vi "Initialise.vi"(8 "error in (no error)":errorcluster, 10 "Message in":refnum<class "InitialiseMessage.lvclass">, 11 "Tomo in":refnum<class "Invivo_Tomo.lvclass">) -> (0 "error out":errorcluster, 3 "Tomo out":refnum<class "Invivo_Tomo.lvclass">)   [LabVIEW 2012, in "Invivo_Tomo.lvclass"]
doc: "This method is called when an initialise message is received. It mainly initialises the RabbitMQ connectivity. \n\nOverride this method when your component needs special initialisation (e.g. of software or hardware resources). In that case, don't forget to call the parent for proper implementation. If your component owns subcomponents, they count as resources, so you have to initialise them by calling their own initialise functions"
uses:
  Invivo_Tomo.lvclass
  <vilib>/Distrio/Murmex/InitialiseMessage/InitialiseMessage.lvclass
  <vilib>/Distrio/Murmex/Murmex/Murmex.lvclass
  Current activity.ctl
panel:
  # "This method is called when the INTIALISE\ntrigger is sent. \n\nOverride this method when your component needs to\nrespond to this trigger. \n\nCall parent for proper implementation"
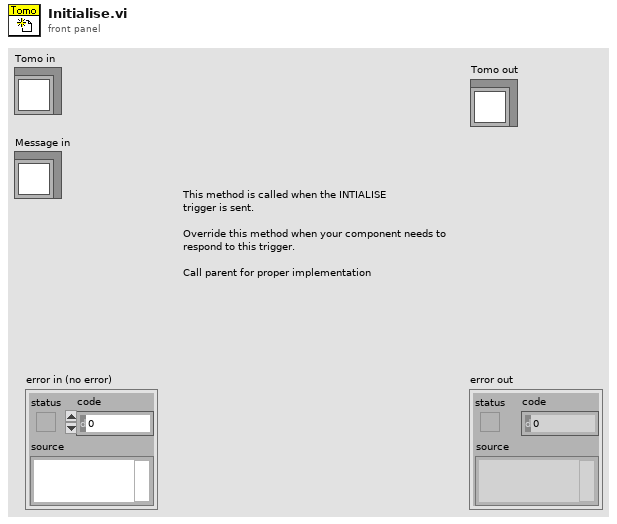
[diagram p1: front panel]
types:
  T1 = typedef "Invivo_Tomo.lvclass/Current activity.ctl" = enum16{"Idle", "Inter-stack motion", "Autofocus", "Stack acquisition"}
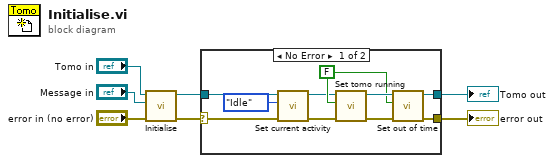
[diagram p0: block diagram]
diagram:
  n1 = call-parent "Initialise.vi"("error in (no error)"="error in (no error)", "Message in"="Message in", "Murmex in"="Tomo in") -> ("error out"=w4:errorcluster, "Murmex out"=w3:refnum<class "Invivo_Tomo.lvclass">)  [unwired: 7 in]
  n2 = case shown="No Error" w4 {
    selector: w4 -> [w10 w18]
    tunnel: w3 -> [w9 w19]
    tunnel: [w16 w18] -> w2
    tunnel: [w14 w19] -> w1
    frame No Error {
      w13 = FALSE ("is acquiring?")
      n3 = call-dynamic "Set current activity.vi"("error in (no error)"=w10, "Current activity"=Current_activity."Idle", "Tomo in"=w9) -> ("error out"=w12:errorcluster, "Tomo out"=w11:refnum<class "Invivo_Tomo.lvclass">)  [unwired: 7 in]
      n4 = call-dynamic "Set tomo running.vi"("error in (no error)"=w12, "tomo running?"=w13, "Tomo in"=w11) -> ("error out"=w17:errorcluster, "Tomo out"=w15:refnum<class "Invivo_Tomo.lvclass">)  [unwired: 7 in]
      n5 = call-dynamic "Set out of time.vi"("error in (no error)"=w17, "out of time?"=w13, "Tomo in"=w15) -> ("error out"=w16:errorcluster, "Tomo out"=w14:refnum<class "Invivo_Tomo.lvclass">)  [unwired: 7 in]
    }
    frame Error {
    }
  }
  "error out" <- w2
  "Tomo out" <- w1
